vi "sandtetris.vi"() -> ()   [LabVIEW 2025]
uses:
  sandtetris_type.ctl
  next_piece.ctl
  <vilib>/sound2/lvsound2.llb/Sound Output Task ID.ctl
  <vilib>/picture/picture.llb/Draw True-Color Pixmap.vi
  <vilib>/sound2/lvsound2.llb/Sound Output Set Volume (Single).vi
  <vilib>/sound2/lvsound2.llb/Sound Output Write (DBL).vi
panel:
  in  "Python Version":string="3.9"
  out "task ID":T1 format="%.0x"
  in  "Music Volume":dbl(slide) scale=0.0..100.0
  out "win":bool
  out "my name":string caption="Your Name (Display Name)"
  out "SandtrisRemote session":refnum<k35>
  out "SandtrisRemote Obj":refnum<k38>
  out "multiplayer":bool
  out "Other":cluster{"Table":picture, "Score":string} caption="demo player"
  in  "join multiplayer":bool
  out "End":bool
  in  "Start":bool
  in  "Hardness":u16(ring) items=["Choose the Hardness", "Easy", "Normal", "Hard"]
  in  "AI Mode":bool
  out "ticker 1":u64
  out "ticker 2":u64
  out "You":T2
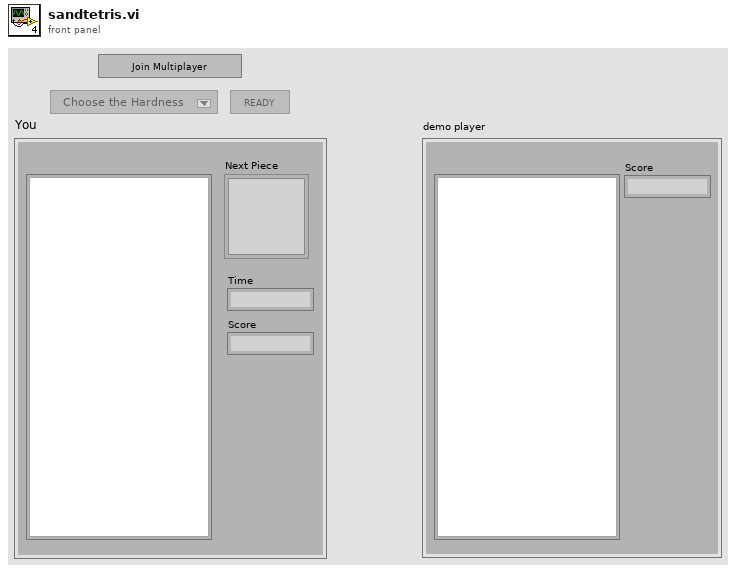
[diagram p1: front panel]
types:
  T1 = typedef "Sound Output Task ID.ctl" = u32
  T2 = typedef "sandtetris_type.ctl" = cluster{"Score":string, "Table":picture, "Time":string, "Next Piece":T3}
  T3 = typedef "next_piece.ctl" = u16
  T4 = enum8{"Enabled", "Disabled", "Disabled and Grayed Out"}
  T5 = cluster{"score":i32, "play_time":string, "next_piece":u16, "game_over":bool}
  T6 = typedef "eventvkey.ctl" = enum16{"ASCII", "Enter", "Return", "Shift", "Ctrl", "Alt", "Cmd", "Opt", "Caps", "NumLock", "Clear", "Break", "Up", "Down", "Left", "Right", "Insert", "Delete", "Home", "End", "PageUp", "PageDown", "Escape", "Help", "Pause", "ScrollLock", "F1", "F2", "F3", "F4", "F5", "F6", "F7", "F8", "F9", "F10", "F11", "F12", "F13", "F14", "F15", "F16", "F17", "F18", "F19", "F20", "F21", "F22", "F23", "F24", "Play", "VolumeUp", "VolumeDown", "Mute", "Two Byte Char"}
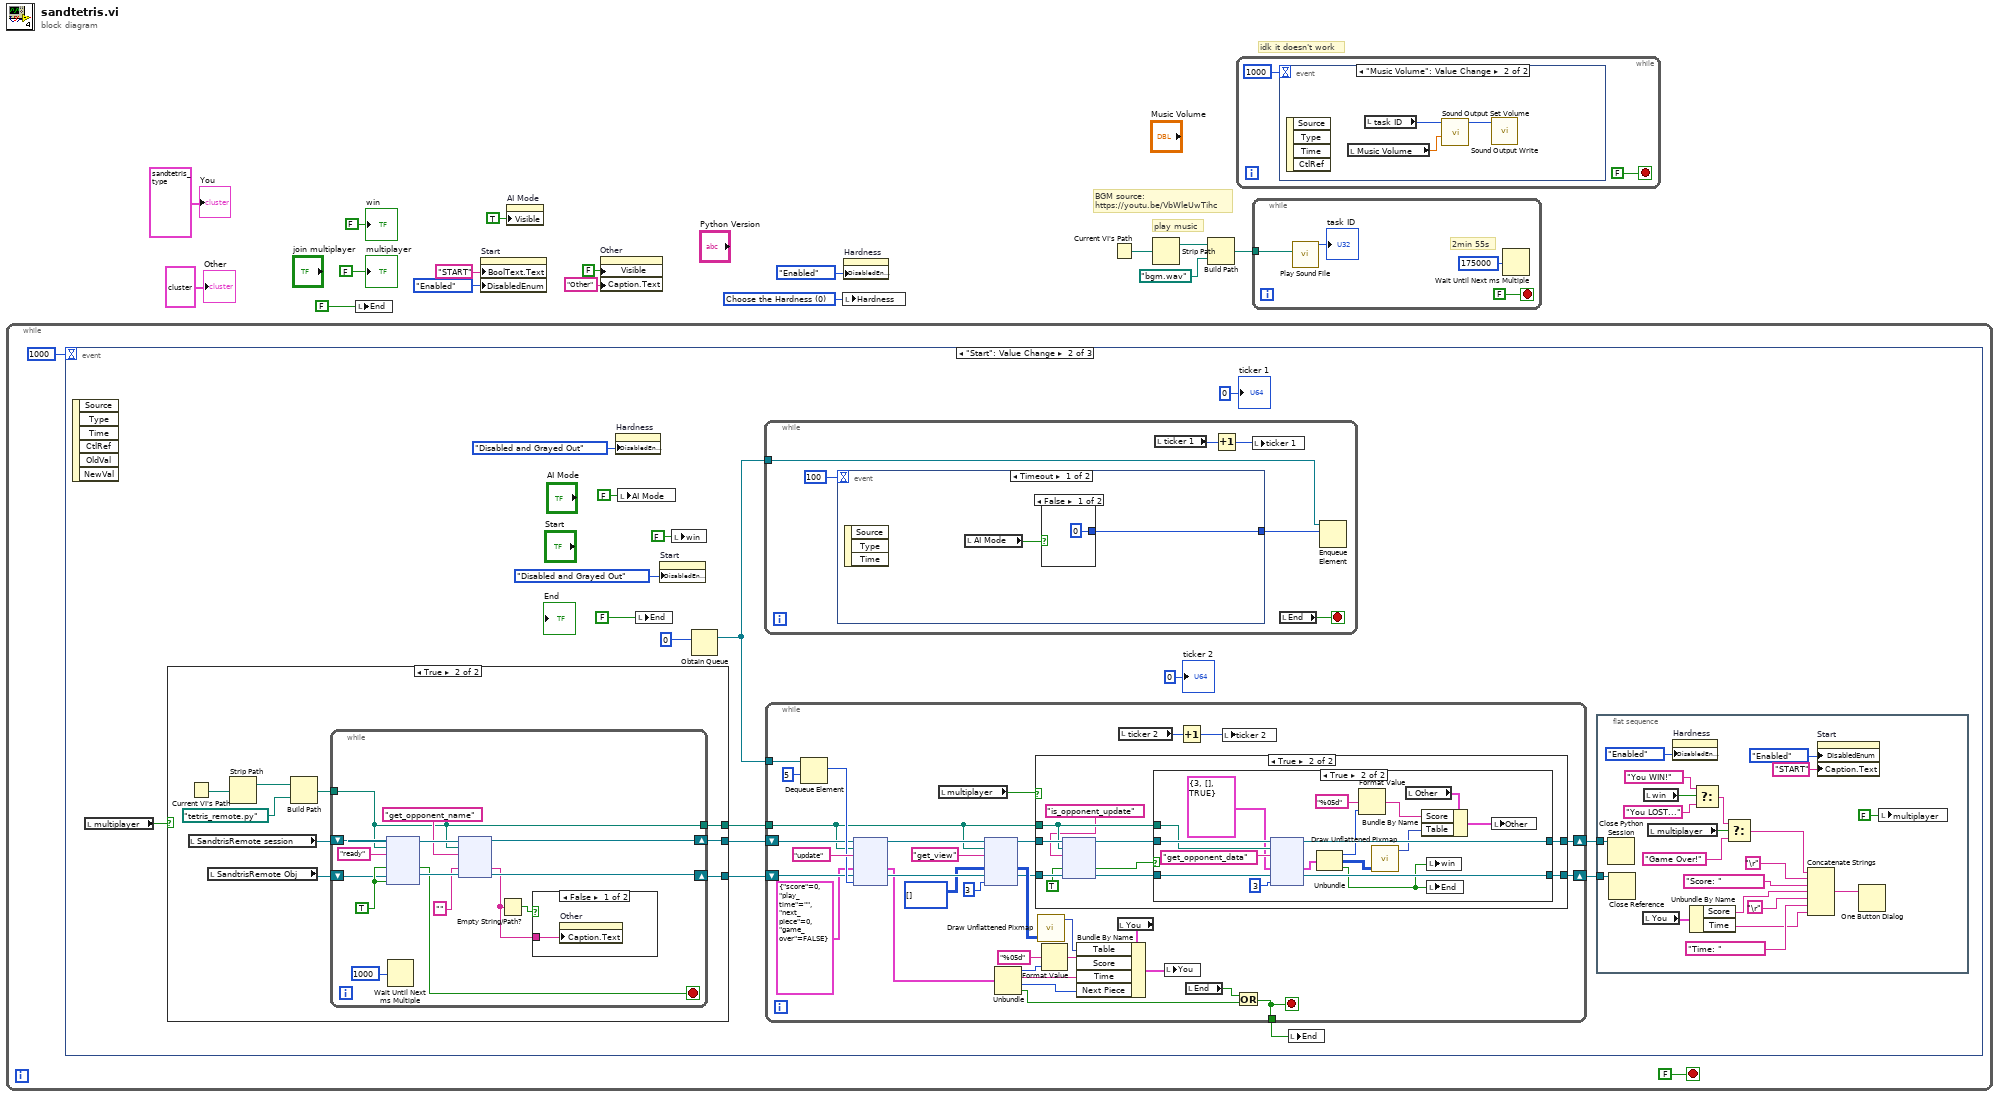
[diagram p0: block diagram]
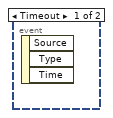
[diagram p2: hidden frame]
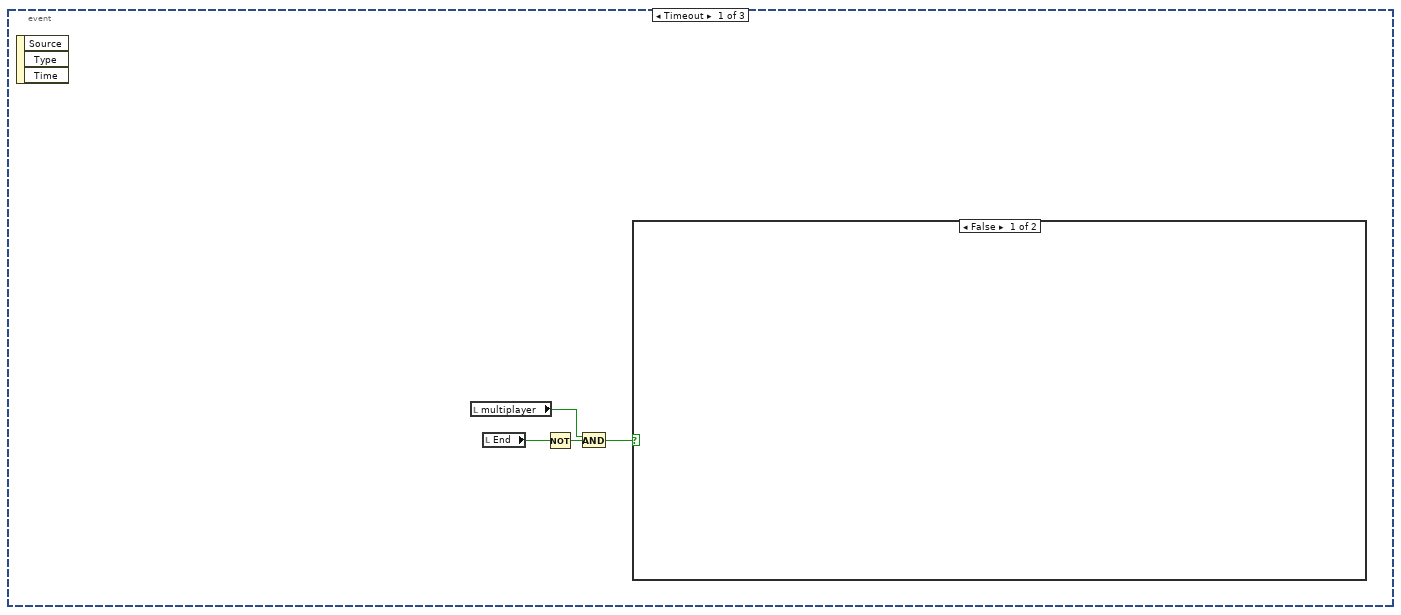
[diagram p3: hidden frame]
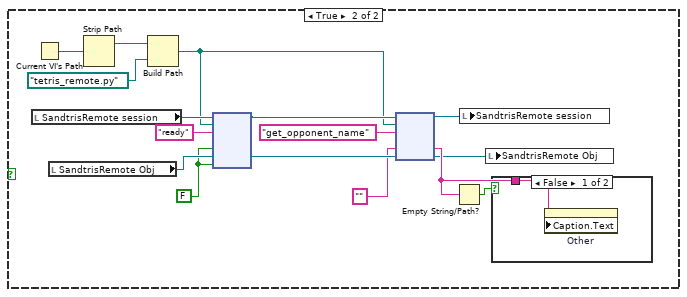
[diagram p4: hidden frame]
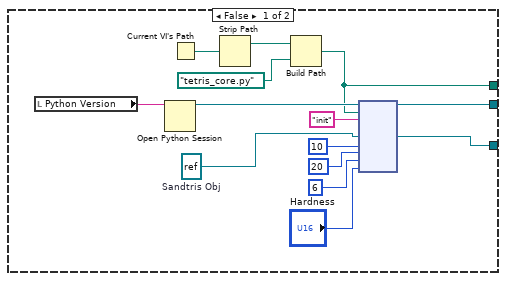
[diagram p6: hidden frame]
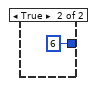
[diagram p10: hidden frame]
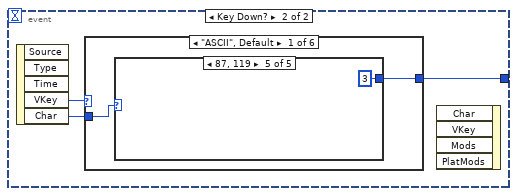
[diagram p11: hidden frame]
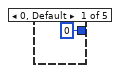
[diagram p12: hidden frame]
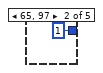
[diagram p13: hidden frame]
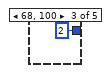
[diagram p14: hidden frame]
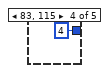
[diagram p15: hidden frame]
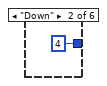
[diagram p16: hidden frame]
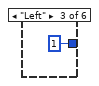
[diagram p17: hidden frame]
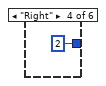
[diagram p18: hidden frame]
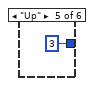
[diagram p19: hidden frame]
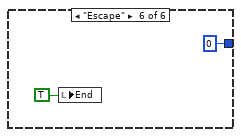
[diagram p20: hidden frame]
diagram:
  w10 = u16 0 items=["Choose the Hardness", "Easy", "Normal", "Hard"] ("Hardness")
  # "BGM source:\nhttps://youtu.be/VbWleUwTihc"
  # "idk it doesn't work"
  # "play music"
  n1 = while {
    stop <- FALSE stop-if-true
    n2 = event shown="[1] \"Start\": Value Change" {
      selector: _ -> [_ _ _]
      dyn-events: _ -> [_ _ _]
      timeout: 1000 -> [_ _ _]
      event Timeout {
        n3 = event-data() -> ()  [unwired: 1 in, 3 out]
        n4 = local read "multiplayer"() -> (w20:bool)
        n5 = local read "End"() -> (w21:bool)
        n6 = Not(x=w21) -> (.not. x?=w22:bool)
        n7 = And(x=w20, y=w22) -> (x .and. y?=w19:bool)
        n8 = case shown="False" w19 {
          frame False {
          }
          frame True {
            w32 = FALSE
            n9 = local read "SandtrisRemote session"() -> (w35:refnum<k35>)
            n10 = Current VI's Path() -> (path=w37:path)
            n11 = local read "SandtrisRemote Obj"() -> (w33:refnum<k38>)
            n12 = Strip Path(path=w37) -> (stripped path=w38:path)  [unwired: 1 out]
            n13 = Build Path(base path=w38, name or relative path=path "tetris_remote.py" ("module path")) -> (appended path=w29:path)
            n14 = node(w35, w29, "ready" ("function name"), w32, w33, w32) -> (w30:refnum<k35>, w28:refnum<k38>)  [unwired: 3 in, 3 out]
            n15 = node(w30, w29, "get_opponent_name" ("function name"), "", w28) -> (w23:refnum<k35>, w25:string, w24:refnum<k38>)  [unwired: 1 in, 3 out]
            n16 = Empty String/Path?(string/path=w25) -> (empty?=w26:bool)
            n17 = local write "SandtrisRemote session"(w23) -> ()
            n18 = local write "SandtrisRemote Obj"(w24) -> ()
            n19 = case shown="False" w26 {
              tunnel: w25 -> [w39 _]
              frame False {
                n20 = property on="Other" class="Clust (strict)"("Caption.Text"=w39) -> ()  [unwired: 2 in, 2 out]
              }
              frame True {
              }
            }
          }
        }
      }
      event "Start": Value Change {
        n21 = event-data() -> ()  [unwired: 1 in, 6 out]
        n22 = local read "multiplayer"() -> (w46:bool)
        n23 = case shown="True" w46 {
          tunnel: [w59 w70] -> w45
          tunnel: [w58 w72] -> w44
          tunnel: [w57 w71] -> w43
          frame False {
            w63 = refnum<k38> refnum  # Sandtris Obj
            n24 = local read "Python Version"() -> (w56:string)
            n25 = Open Python Session(python version=w56) -> (session out=w69:refnum<k35>)  [unwired: 2 in, 1 out]
            n26 = Current VI's Path() -> (path=w68:path)
            n27 = Strip Path(path=w68) -> (stripped path=w67:path)  [unwired: 1 out]
            n28 = Build Path(base path=w67, name or relative path=path "tetris_core.py" ("module path")) -> (appended path=w59:path)
            n29 = node(w69, w59, "init" ("function name"), w63, 10, 20, 6, "Hardness") -> (w57:refnum<k35>, w58:refnum<k38>)  [unwired: 5 in, 3 out]
          }
          frame True {
            n30 = Current VI's Path() -> (path=w78:path)
            n31 = local read "SandtrisRemote session"() -> (w74:refnum<k35>)
            n32 = local read "SandtrisRemote Obj"() -> (w73:refnum<k38>)
            n33 = Strip Path(path=w78) -> (stripped path=w77:path)  [unwired: 1 out]
            n34 = Build Path(base path=w77, name or relative path=path "tetris_remote.py" ("module path")) -> (appended path=w75:path)
            n35 = while {
              tunnel: w75 -> [w81]
              shift-right: [w82] -> w71
              shift-left: w74 -> [w85]
              shift-right: [w83] -> w72
              shift-left: w73 -> [w84]
              tunnel: [w81] -> w70
              stop <- w87 stop-if-true
              w88 = TRUE
              n36 = node(w85, w81, "ready" ("function name"), w88, w84, w88) -> (w93:refnum<k35>, w87:bool, w92:refnum<k38>)  [unwired: 2 in, 3 out]
              n37 = Wait Until Next ms Multiple(millisecond multiple=u32 1000) -> ()  [unwired: 1 out]
              n38 = node(w93, w81, "get_opponent_name" ("function name"), "", w92) -> (w82:refnum<k35>, w79:string, w83:refnum<k38>)  [unwired: 1 in, 3 out]
              n39 = Empty String/Path?(string/path=w79) -> (empty?=w80:bool)
              n40 = case shown="False" w80 {
                tunnel: w79 -> [w94 _]
                frame False {
                  n41 = property on="Other" class="Clust (strict)"("Caption.Text"=w94) -> ()  [unwired: 2 in, 2 out]
                }
                frame True {
                }
              }
            }
          }
        }
        n42 = property on="Hardness" class="Ring (strict)"("DisabledEnum"=T4."Disabled and Grayed Out" ("Disabled")) -> ()  [unwired: 2 in, 2 out]
        n43 = local write "AI Mode"(FALSE ("AI Mode")) -> ()
        n44 = local write "End"(FALSE ("End")) -> ()
        n45 = property on="Start" class="Bool"("DisabledEnum"=T4."Disabled and Grayed Out" ("Disabled")) -> ()  [unwired: 2 in, 2 out]
        n46 = local write "win"(FALSE ("win")) -> ()
        n47 = Obtain Queue(element data type=u16 0) -> (queue out=w55:refnum<queue>)  [unwired: 4 in, 2 out]
        n48 = while {
          tunnel: w55 -> [w184]
          stop <- w180 stop-if-true
          n49 = event shown="[0] Timeout" {
            selector: _ -> [_ _]
            dyn-events: _ -> [_ _]
            timeout: 100 -> [_ _]
            tunnel: [w187 w191] -> w183
            event Timeout {
              n50 = event-data() -> ()  [unwired: 1 in, 3 out]
              n51 = local read "AI Mode"() -> (w186:bool)
              n52 = case shown="False" w186 {
                tunnel: [u16 0 ("element") u16 6 ("element")] -> w187
                frame False {
                }
                frame True {
                }
              }
            }
            event Key Down? {
              n53 = event-data() -> ("VKey"=w192:T6, "Char"=w190:i16)  [unwired: 1 in, 3 out]
              n54 = case shown="\"ASCII\", Default" w192 {
                tunnel: [w193 u16 4 ("element") u16 1 ("element") u16 2 ("element") u16 3 ("element") u16 0 ("element")] -> w191
                tunnel: w190 -> [w194 _ _ _ _ _]
                frame "ASCII", Default {
                  n55 = case shown="87, 119" w194 {
                    tunnel: [u16 0 ("element") u16 1 ("element") u16 2 ("element") u16 4 ("element") u16 3 ("element")] -> w193
                    frame 0, Default {
                    }
                    frame 65, 97 {
                    }
                    frame 68, 100 {
                    }
                    frame 83, 115 {
                    }
                    frame 87, 119 {
                    }
                  }
                }
                frame "Down" {
                }
                frame "Left" {
                }
                frame "Right" {
                }
                frame "Up" {
                }
                frame "Escape" {
                  n56 = local write "End"(TRUE ("End")) -> ()
                }
              }
              n57 = event-data() -> ()  [unwired: 5 in, 1 out]
            }
          }
          n58 = local read "ticker 1"() -> (w182:u64)
          n59 = Increment(x=w182) -> (x+1=w181:u64)
          n60 = local write "ticker 1"(w181) -> ()
          n61 = local read "End"() -> (w180:bool)
          n62 = Enqueue Element(queue=w184, element=w183) -> ()  [unwired: 2 in, 3 out]
        }
        n63 = while {
          tunnel: w55 -> [w148]
          tunnel: w45 -> [w117]
          shift-right: [w121] -> w49
          shift-left: w43 -> [w141]
          shift-right: [w119] -> w48
          shift-left: w44 -> [w140]
          tunnel: [w116] -> w41
          stop <- w116 stop-if-true
          n64 = Dequeue Element(queue=w148, timeout in ms (-1)=5) -> (element=w144:u16)  [unwired: 1 in, 3 out]
          n65 = node(w141, w117, "update" ("function name"), T5 {"score"=0, "play_time"="", "next_piece"=0, "game_over"=FALSE}, w140, w144) -> (w147:refnum<k35>, w130:T5, w143:refnum<k38>)  [unwired: 2 in, 3 out]
          n66 = local read "multiplayer"() -> (w122:bool)
          n67 = node(w147, w117, "get_view" ("function name"), u32[][] [], w143, 3) -> (w120:refnum<k35>, w139:u32[][], w118:refnum<k38>)  [unwired: 2 in, 3 out]
          n68 = Unbundle(w130) -> ("score"=w129:i32, "play_time"=w126:string, "next_piece"=w125:u16, "game_over"=w124:bool)
          n69 = case shown="True" w122 {
            tunnel: [w150 w152] -> w121
            tunnel: w120 -> [w150 w160]
            tunnel: [w149 w151] -> w119
            tunnel: w118 -> [w149 w158]
            tunnel: w117 -> [_ w156]
            frame False {
            }
            frame True {
              n70 = node(w160, w156, "is_opponent_update" ("function name"), TRUE, w158) -> (w159:refnum<k35>, w153:bool, w157:refnum<k38>)  [unwired: 1 in, 3 out]
              n71 = case shown="True" w153 {
                tunnel: w159 -> [w162 w179]
                tunnel: w157 -> [w161 w178]
                tunnel: w156 -> [_ w177]
                tunnel: [w162 w175] -> w152
                tunnel: [w161 w174] -> w151
                frame False {
                }
                frame True {
                  n72 = node(w179, w177, "get_opponent_data" ("function name"), cluster{i32, u32[][], bool} {3, [], TRUE} ("Other"), w178, 3) -> (w175:refnum<k35>, w171:cluster{i32, u32[][], bool}, w174:refnum<k38>)  [unwired: 2 in, 3 out]
                  n73 = Unbundle(w171) -> (w169:i32, w170:u32[][], w164:bool)
                  n74 = Format Value(format string="%05d", value (0)=w169) -> (output string=w167:string)  [unwired: 1 in]
                  n75 = call-poly <vilib>:"Draw Unflattened Pixmap.vi"("data (RGB format)"=w170) -> ("new picture"=w166:picture)  [unwired: 8 in]
                  n76 = local read "Other"() -> (w168:cluster{"Table":picture, "Score":string})
                  n77 = Bundle By Name(cluster=w168, "Score"=w167, "Table"=w166) -> (w165:cluster{"Table":picture, "Score":string})
                  n78 = local write "win"(w164) -> ()
                  n79 = local write "End"(w164) -> ()
                  n80 = local write "Other"(w165) -> ()
                }
              }
            }
          }
          n81 = call-poly <vilib>:"Draw Unflattened Pixmap.vi"("data (RGB format)"=w139) -> ("new picture"=w136:picture)  [unwired: 8 in]
          n82 = Format Value(format string="%05d", value (0)=w129) -> (output string=w128:string)  [unwired: 1 in]
          n83 = local read "You"() -> (w138:T2)
          n84 = Bundle By Name(cluster=w138, "Table"=w136, "Score"=w128, "Time"=w126, "Next Piece"=w125) -> (w137:T2)
          n85 = local read "ticker 2"() -> (w142:u64)
          n86 = local write "You"(w137) -> ()
          n87 = Increment(x=w142) -> (x+1=w134:u64)
          n88 = local read "End"() -> (w123:bool)
          n89 = local write "ticker 2"(w134) -> ()
          n90 = Or(x=w123, y=w124) -> (x .or. y?=w116:bool)
        }
        n91 = local write "End"(w41) -> ()
        n92 = flat-sequence {
          tunnel: w49 -> [w115]
          tunnel: w48 -> [w114]
          frame #0 {
            n93 = Close Python Session(session in=w115) -> ()  [unwired: 1 in, 1 out]
            n94 = Close Reference(reference=w114) -> ()  [unwired: 1 in, 1 out]
            n95 = local read "You"() -> (w113:T2)
            n96 = local read "win"() -> (w100:bool)
            n97 = local read "multiplayer"() -> (w103:bool)
            n98 = property on="Hardness" class="Ring (strict)"("DisabledEnum"=T4."Enabled" ("Disabled")) -> ()  [unwired: 2 in, 2 out]
            n99 = Unbundle By Name(w113) -> ("Score"=w112:string, "Time"=w107:string)
            n100 = Select(t="You WIN!", s=w100, f="You LOST...") -> (s? t:f=w101:string)
            n101 = Select(t=w101, s=w103, f="Game Over!") -> (s? t:f=w97:string)
            n102 = Concatenate Strings(w97, "\r", "Score: ", w112, "\r", "Time: ", w107) -> (w106:string)
            n103 = property on="Start" class="Bool"("DisabledEnum"=T4."Enabled" ("Disabled"), "Caption.Text"="START") -> ()  [unwired: 2 in, 2 out]
            n104 = One Button Dialog(message=w106) -> ()  [unwired: 1 in, 1 out]
            n105 = local write "multiplayer"(FALSE ("multiplayer")) -> ()
          }
        }
        "ticker 2" <- u64 0 ("tick2")
        "ticker 1" <- u64 0 ("tick1")
      }
      event "join multiplayer": Value Change {
        n106 = event-data() -> ()  [unwired: 1 in, 6 out]
        n107 = local read "Python Version"() -> (w206:string)
        n108 = Current VI's Path() -> (path=w215:path)
        n109 = Open Python Session(python version=w206) -> (session out=w213:refnum<k35>)  [unwired: 2 in, 1 out]
        n110 = Strip Path(path=w215) -> (stripped path=w216:path)  [unwired: 1 out]
        n111 = local write "join multiplayer"(FALSE ("join multiplayer")) -> ()
        n112 = Build Path(base path=w216, name or relative path=path "tetris_remote.py" ("module path")) -> (appended path=w212:path)
        n113 = while {
          tunnel: w213 -> [w251]
          tunnel: w212 -> [w231]
          shift-right: [w240] -> w210
          shift-left: _ -> [_]
          tunnel: [w236] -> w208
          tunnel: [w232] -> w211
          tunnel: [w231] -> w207
          stop <- w238 stop-if-true
          w249 = refnum<k38> refnum  # Sandtris Remote Obj
          n114 = call "Join Server"("Enable"=TRUE) -> ("Your Name (Display Name)"=w243:string, "Server IP"=w244:string, "OK"=w232:bool)  [unwired: 15 in, 1 out]
          "my name" <- w243
          n115 = node(w251, w231, "init" ("function name"), w249, 10, 20, 6, w244, w243) -> (w237:refnum<k35>, w241:refnum<k38>)  [unwired: 6 in, 3 out]
          n116 = node(w237, w231, "join" ("function name"), 0, w241) -> (w236:refnum<k35>, w235:i32, w240:refnum<k38>)  [unwired: 1 in, 3 out]
          n117 = Select(t=w235, s=w232, f=0) -> (s? t:f=w234:i32)
          n118 = case shown="4" w234 {
            tunnel: [TRUE FALSE FALSE FALSE FALSE] -> w238
            frame 0 {
            }
            frame 1, Default {
              n119 = One Button Dialog(message="Cannot connect to server. Please try again later.") -> ()  [unwired: 1 in, 1 out]
            }
            frame 2 {
              n120 = One Button Dialog(message="The server is full!") -> ()  [unwired: 1 in, 1 out]
            }
            frame 3 {
              n121 = One Button Dialog(message="Your name has already taken, please change another one.") -> ()  [unwired: 1 in, 1 out]
            }
            frame 4 {
              n122 = One Button Dialog(message="Invalid name! Please avoid using non-alphanumeric characters!") -> ()  [unwired: 1 in, 1 out]
            }
          }
        }
        n123 = case shown="True" w211 {
          tunnel: w210 -> [_ w221]
          tunnel: w208 -> [_ w223]
          tunnel: w207 -> [_ w218]
          frame False {
          }
          frame True {
            n124 = local write "multiplayer"(TRUE ("multiplayer")) -> ()
            n125 = property on="Start" class="Bool"("BoolText.Text"="READY" ("Boolean Text.Text")) -> ()  [unwired: 2 in, 2 out]
            n126 = node(w223, w218, "get_hardness" ("function name"), 0, w221) -> (→"SandtrisRemote session":refnum<k35>, w219:i32, →"SandtrisRemote Obj":refnum<k38>)  [unwired: 1 in, 3 out]
            n127 = local write "Hardness"(w219) -> ()
            n128 = property on="Other" class="Clust (strict)"("Visible"=TRUE, "Caption.Text"="Waiting for another player..." ("Label.Text")) -> ()  [unwired: 2 in, 2 out]
            n129 = property on="Hardness" class="Ring (strict)"("DisabledEnum"=T4."Disabled and Grayed Out" ("Disabled")) -> ()  [unwired: 2 in, 2 out]
            n130 = property on="AI Mode" class="Bool (strict)"("Visible"=FALSE) -> ()  [unwired: 2 in, 2 out]
          }
        }
      }
    }
  }
  n131 = local write "End"(FALSE ("End")) -> ()
  n132 = property on="Start" class="Bool"("BoolText.Text"="START" ("Boolean Text.Text"), "DisabledEnum"=T4."Enabled" ("Disabled")) -> ()  [unwired: 2 in, 2 out]
  n133 = property on="AI Mode" class="Bool (strict)"("Visible"=TRUE) -> ()  [unwired: 2 in, 2 out]
  n134 = property on="Other" class="Clust (strict)"("Visible"=FALSE, "Caption.Text"="Other" ("Label.Text")) -> ()  [unwired: 2 in, 2 out]
  n135 = local write "Hardness"(w10) -> ()
  n136 = property on="Hardness" class="Ring (strict)"("DisabledEnum"=T4."Enabled" ("Disabled")) -> ()  [unwired: 2 in, 2 out]
  n137 = Current VI's Path() -> (path=w3:path)
  n138 = Strip Path(path=w3) -> (stripped path=w4:path)  [unwired: 1 out]
  n139 = Build Path(base path=w4, name or relative path=path "bgm.wav" ("module path")) -> (appended path=w1:path)
  n140 = while {
    stop <- FALSE stop-if-true
    n141 = event shown="[1] \"Music Volume\": Value Change" {
      selector: _ -> [_ _]
      dyn-events: _ -> [_ _]
      timeout: 1000 -> [_ _]
      event Timeout {
        n142 = event-data() -> ()  [unwired: 1 in, 3 out]
      }
      event "Music Volume": Value Change {
        n143 = event-data() -> ()  [unwired: 1 in, 4 out]
        n144 = local read "Music Volume"() -> (w265:dbl)
        n145 = local read "task ID"() -> (w264:T1)
        n146 = call-poly <vilib>:"Sound Output Set Volume.vi"("volume"=w265, "task ID"=w264) -> ("task ID out"=w263:T1)  [unwired: 8 in, 1 out]
        n147 = call-poly <vilib>:"Sound Output Write.vi"("task ID"=w263) -> ()  [unwired: 9 in, 2 out]
      }
    }
  }
  n148 = while {
    tunnel: w1 -> [w267]
    stop <- FALSE stop-if-true
    # "2min 55s"
    n149 = call <vilib>:"Play Sound File.vi"("path"=w267) -> ("task ID"=→"task ID":T1)  [unwired: 9 in, 1 out]
    n150 = Wait Until Next ms Multiple(millisecond multiple=u32 175000) -> ()  [unwired: 1 out]
  }
  "multiplayer" <- FALSE ("multiplayer")
  "You" <- T2 {"Score"="00000", "Table"=bytes[0], "Time"="00:00", "Next Piece"=0} ("You")
  "Other" <- cluster{"Table":picture, "Score":string} {"Table"=bytes[0], "Score"="0"} ("Other")
  "win" <- FALSE ("win")
